vi "Initialize Front Panel.vi"(8 "error in (no error)":errorcluster, 11 "VerticalSlide In":refnum<class "VerticalSlide.lvclass">) -> (0 "error out":errorcluster, 3 "VerticalSlide Out":refnum<class "VerticalSlide.lvclass">)   [LabVIEW 2020, in "MVAExamples.lvlib" / "VerticalSlide.lvclass"]
doc: "<License>\nCopyright © 2017 Composed Systems, LLC | All rights reserved\nwww.composed.io\n\nAuthor: Ethan Stern <ethan.stern@composed.io>\n\nThis software is provided \"AS IS\" WITHOUT WARRANTIES, either express or implied, AND IS FOR EDUCATIONAL PURPOSES ONLY.\n</License>"
uses:
  VerticalSlide.lvclass
  VerticalSlide.lvclass/VerticalSlide.ctl
  modules/mva-viewable/Source/IViewable/IViewable/IViewable.lvclass
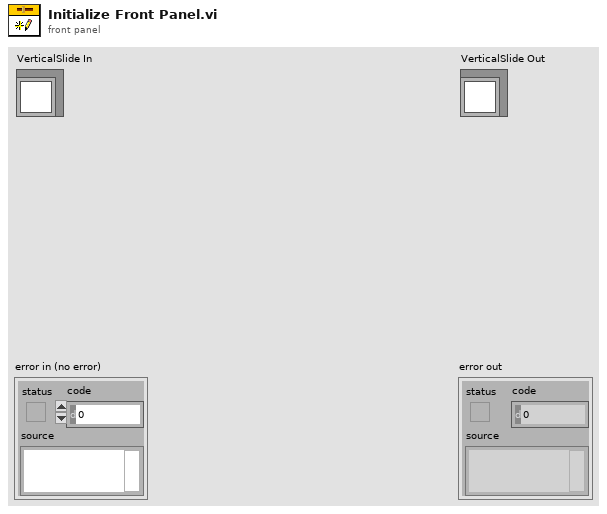
[diagram p1: front panel]
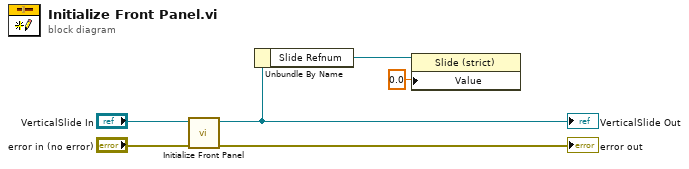
[diagram p0: block diagram]
diagram:
  n1 = call-parent "Initialize Front Panel.vi"("error in (no error)"="error in (no error)", "IViewable in"="VerticalSlide In") -> ("error out"=→"error out":errorcluster, "IViewable out"=w3:refnum<class "VerticalSlide.lvclass">)  [unwired: 8 in]
  "VerticalSlide Out" <- w3
  n2 = Unbundle By Name(w3) -> ("Slide Refnum"=w2:refnum<vi>)
  n3 = property class="Slide (strict)"(reference=w2, "Value"=0.0) -> ()  [unwired: 1 in, 2 out]
